vi "Main_DAQ.vi"() -> ()   [LabVIEW 2018]
uses:
  <vilib>/DAQmx/read.llb/DAQmx Read (Analog 2D DBL NChan NSamp).vi
  <vilib>/Analysis/baseanly.llb/Mean (DBL).vi
  <vilib>/DAQmx/create/channels.llb/DAQmx Create Channel (AI-Voltage-Basic).vi
  <vilib>/DAQmx/configure/timing.llb/DAQmx Timing (Sample Clock).vi
  <vilib>/DAQmx/configure/trigger.llb/DAQmx Start Trigger (Digital Edge).vi
  <vilib>/DAQmx/configure/trigger.llb/DAQmx Start Trigger (Time).vi
  <vilib>/DAQmx/configure/trigger.llb/DAQmx Start Trigger (Analog Edge).vi
  <vilib>/DAQmx/miscellaneous.llb/DAQmx Fill In Error Info.vi
  <resource>/objmgr/daqmx.rc
  <vilib>/Analysis/NI_AALBase.lvlib
panel:
  out "Waveform Graph 2":dbl[][](graph)
  out "Waveform Chart":dbl[](graph)
  in  "length":i32
  in  "Start index":i32
  in  "Path":path
  in  "Name File":string
  in  "SAVE ?":bool
  in  "SENSOR":bool
  in  "Trigger Type":T1(tab)=enum."Digital Start"
  in  "Digital Start Trigger Edge":i32(ring)=10280 caption="Edge" items=["Rising"=10280, "Falling"=10171]
  in  "Digital Start Trigger Source":tag="/Dev2/PFI0" caption="Source"
  in  "Digital Pause Trigger Pause When":i32(ring)=10192 caption="Pause When" items=["High"=10192, "Low"=10214]
  in  "Digital Pause Trigger Source":tag="/Dev1/PFI0" caption="Source"
  in  "Analog Start Trigger Level":dbl caption="Level" format="%0.2f"
  in  "Analog Start Trigger Hysteresis":dbl caption="Hysteresis" format="%.2f"
  in  "Analog Start Trigger Slope":i32(ring)=10280 caption="Slope" items=["Rising"=10280, "Falling"=10171]
  in  "Analog Start Trigger Source":string="APFI0" caption="Source"
  in  "Analog Pause Trigger Source":string="APFI0" caption="Source"
  in  "Analog Pause Trigger Pause When":i32(ring)=10093 caption="Pause When" items=["Above Level"=10093, "Below Level"=10107]
  in  "Analog Pause Trigger Level":dbl caption="Level" format="%.2f"
  in  "When":timestamp
  in  "Select Time\nManually":bool
  in  "Number of Samples":i32=100
  in  "Sample Rate":dbl=10000.0
  in  "Sample Clock Source":tag="OnboardClock"
  in  "Terminal Configuration":i32(ring)=10083 items=["default"=-1, "RSE"=10083, "NRSE"=10078, "Differential"=10106, "Pseudodifferential"=12529]
  in  "Max Voltage":dbl=10.0
  in  "Min Voltage":dbl=-10.0
  in  "Physical Channel":tag="Dev2/ai3:4"
  out "Actual Sample Rate":dbl=1000.0 format="%0.2f"
  # "Graph"
  # "Channel Settings"
  # "Control Program"
  # "Timing Settings"
  # "Saving Data Settings"
  # "Trigger Settings"
  # "To enable triggers, select a tab above, and configure the settings.\n\nNot all hardware supports all trigger types. Refer to your device documentation for more information."
  # "This trigger type is not supported in continuous sample timing. \n\nRefer to your device documentation for more information on which triggers are supported."
  # "This trigger type is not supported in continuous sample timing. \n\nRefer to your device documentation for more information on which triggers are supported."
  # "If time is not manually set, task will begin after 10 seconds"
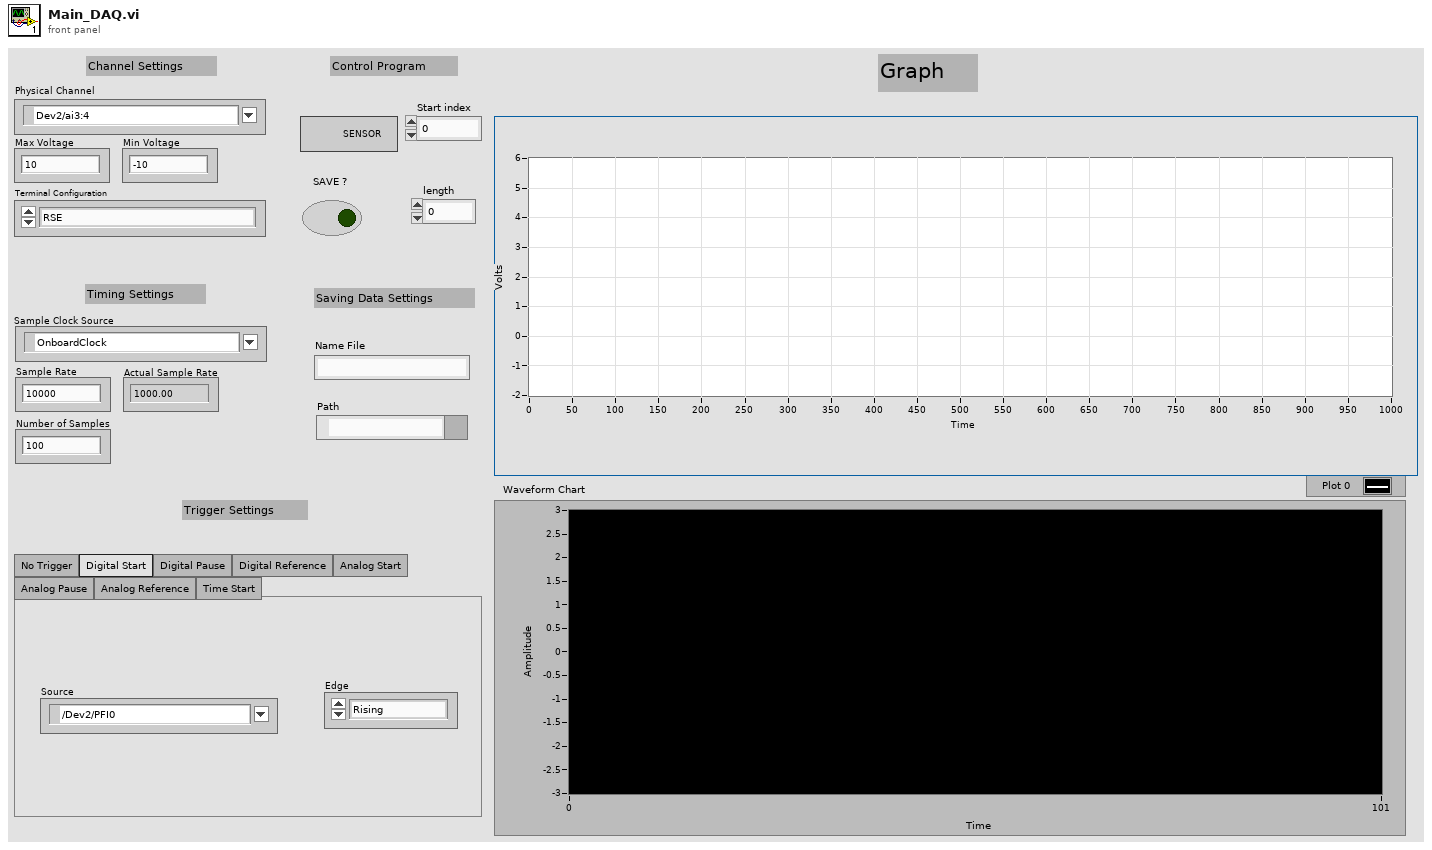
[diagram p1: front panel]
types:
  T1 = enum32{"No Trigger", "Digital Start", "Digital Pause", "Digital Reference", "Analog Start", "Analog Pause", "Analog Reference", "Time Start"}
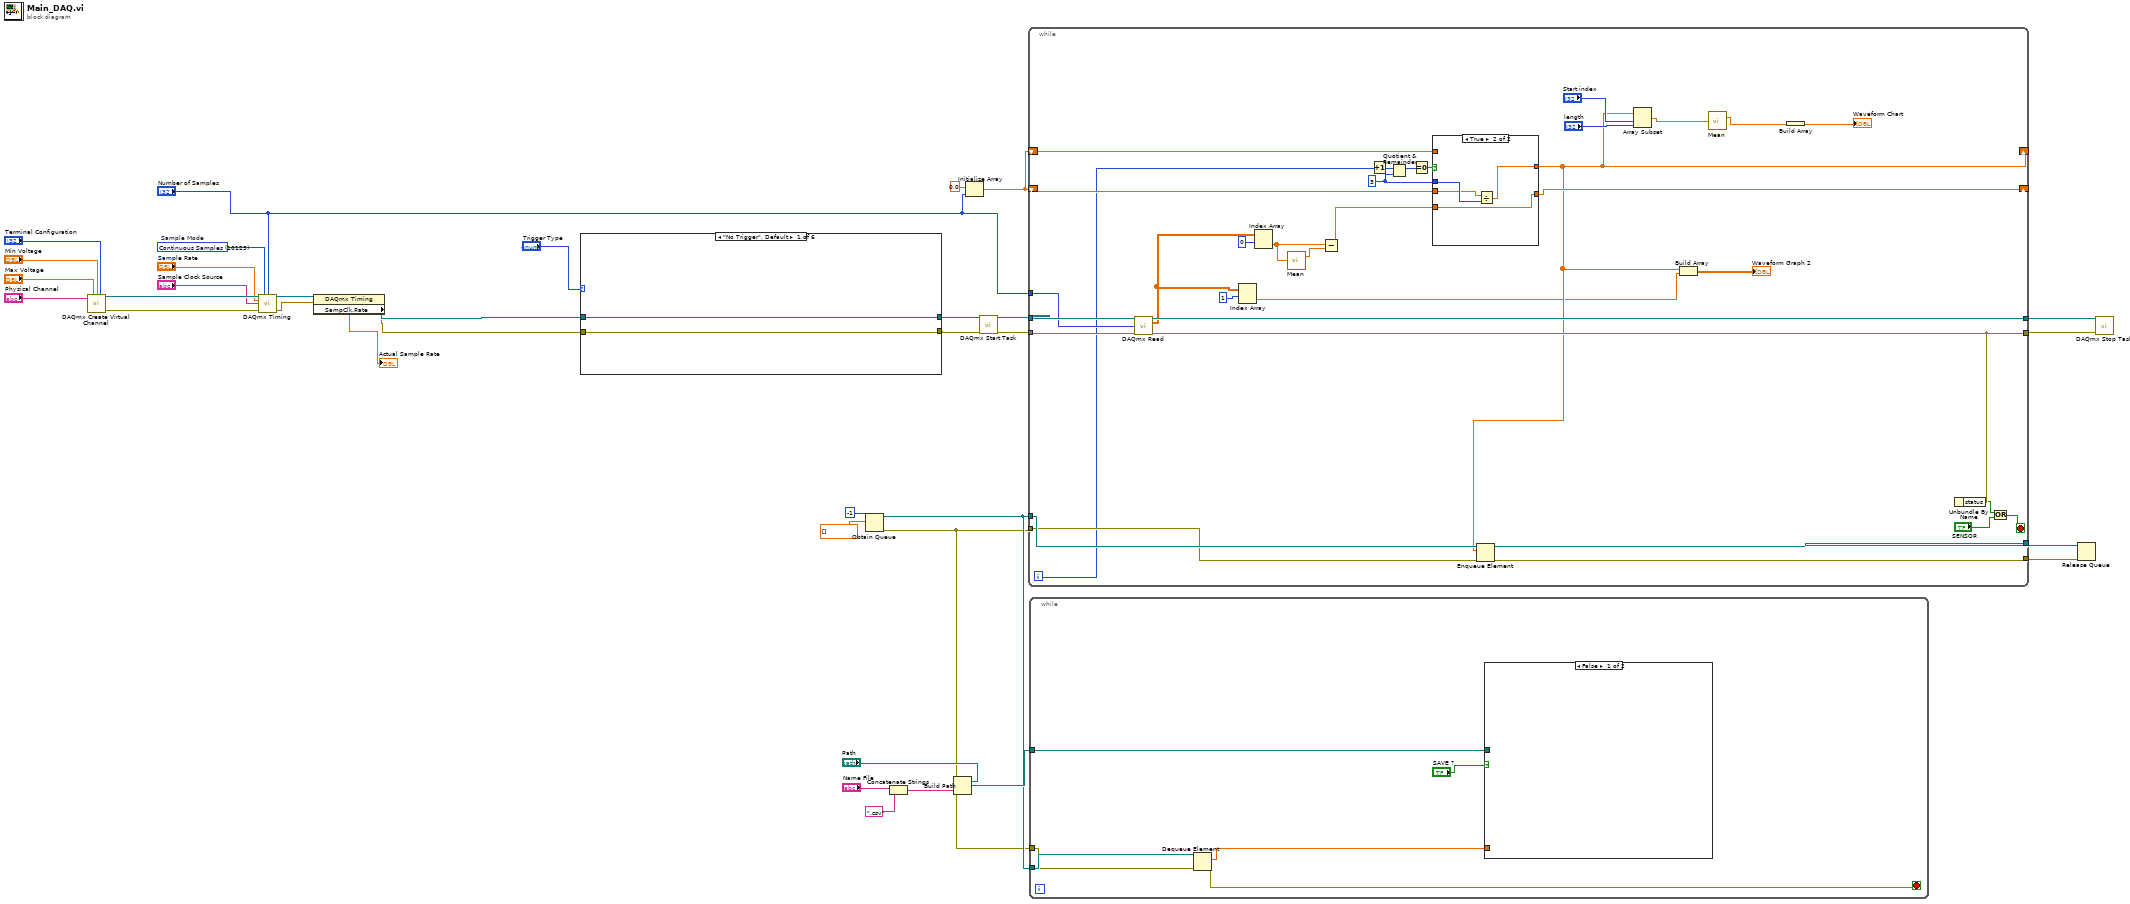
[diagram p0: block diagram]
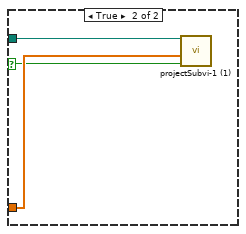
[diagram p2: hidden frame]
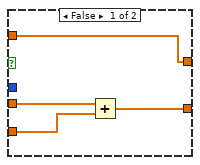
[diagram p3: hidden frame]
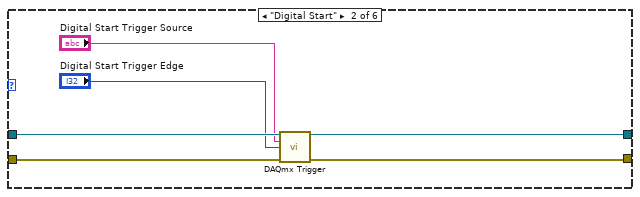
[diagram p4: hidden frame]
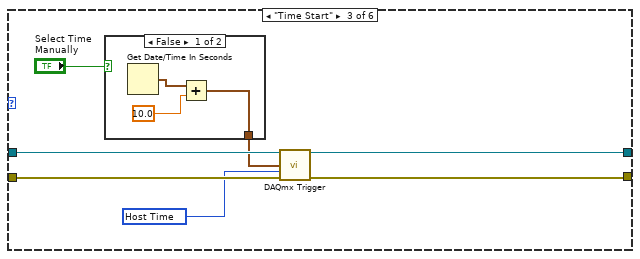
[diagram p5: hidden frame]
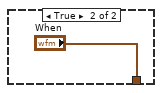
[diagram p6: hidden frame]
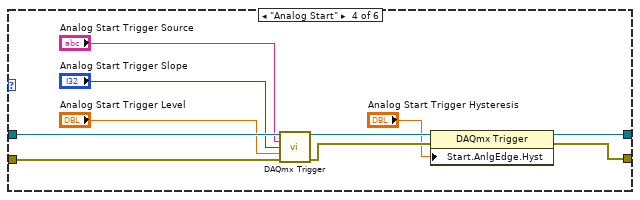
[diagram p7: hidden frame]
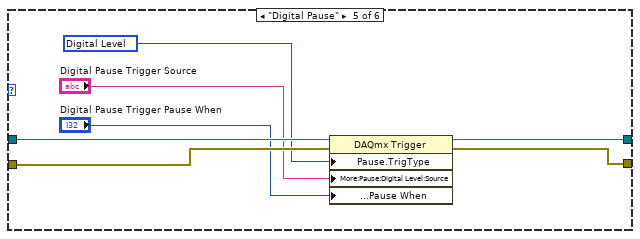
[diagram p8: hidden frame]
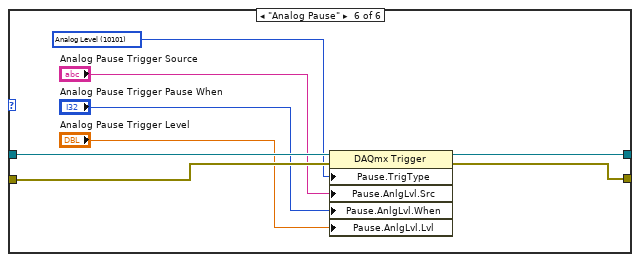
[diagram p9: hidden frame]
diagram:
  w33 = 10123 items=["Finite Samples"=10178, "Continuous Samples"=10123, "Hardware Timed Single Point"=12522]  # Sample Mode
  n1 = call-poly <vilib>:"DAQmx Create Virtual Channel.vi"("maximum value"="Max Voltage", "minimum value"="Min Voltage", "input terminal configuration"="Terminal Configuration", "physical channels"="Physical Channel") -> ("task out"=w31:refnum<k21>, "error out"=w32:errorcluster)  [unwired: 10 in]
  n2 = call-poly <vilib>:"DAQmx Timing.vi"("task/channels in"=w31, "sample mode"=w33, "samples per channel"="Number of Samples", "rate"="Sample Rate", "source"="Sample Clock Source", "error in"=w32) -> ("task out"=w35:refnum<k21>, "error out"=w34:errorcluster)  [unwired: 8 in]
  n3 = property class="DAQmx Timing"(reference=w35, error in=w34) -> (reference out=w20:refnum<k21>, error out=w19:errorcluster, "SampClk.Rate"=→"Actual Sample Rate":dbl)
  n4 = case shown="\"No Trigger\", Default" "Trigger Type" {
    tunnel: w20 -> [w37 w43 w50 w64 w71 w79]
    tunnel: w19 -> [w36 w42 w49 w63 w68 w76]
    tunnel: [w37 w41 w48 w61 w70 w78] -> w21
    tunnel: [w36 w40 w47 w60 w69 w77] -> w22
    frame "No Trigger", Default {
    }
    frame "Digital Start" {
      n5 = call-poly <vilib>:"DAQmx Trigger.vi"("task/channels in"=w43, "source"="Digital Start Trigger Source", "edge"="Digital Start Trigger Edge", "error in"=w42) -> ("task out"=w41:refnum<k21>, "error out"=w40:errorcluster)  [unwired: 10 in]
    }
    frame "Time Start" {
      w46 = 16126 items=["Host Time"=16126, "I/O Device Time"=16127] ("timescale")
      n6 = case shown="False" "Select Time\nManually" {
        tunnel: [w51 "When"] -> w44
        frame False {
          n7 = Get Date/Time In Seconds() -> (seconds since 1Jan1904=w53:timestamp)
          n8 = Add(x=w53, y=10.0) -> (x+y=w51:timestamp)
        }
        frame True {
        }
      }
      n9 = call-poly <vilib>:"DAQmx Trigger.vi"("task/channels in"=w50, "when"=w44, "timescale"=w46, "error in"=w49) -> ("task out"=w48:refnum<k21>, "error out"=w47:errorcluster)  [unwired: 10 in]
    }
    frame "Analog Start" {
      n10 = call-poly <vilib>:"DAQmx Trigger.vi"("task/channels in"=w64, "source"="Analog Start Trigger Source", "slope"="Analog Start Trigger Slope", "level"="Analog Start Trigger Level", "error in"=w63) -> ("task out"=w59:refnum<k21>, "error out"=w58:errorcluster)  [unwired: 9 in]
      n11 = property class="DAQmx Trigger"(reference=w59, error in=w58, "Start.AnlgEdge.Hyst"="Analog Start Trigger Hysteresis") -> (reference out=w61:refnum<k21>, error out=w60:errorcluster)
    }
    frame "Digital Pause" {
      w67 = 10152 items=["Analog Level"=10101, "Analog Window"=10103, "Digital Level"=10152, "Digital Pattern"=10398, "None"=10230] ("Pause.TrigType")
      n12 = property class="DAQmx Trigger"(reference=w71, error in=w68, "Pause.TrigType"=w67, "More:Pause:Digital Level:Source"="Digital Pause Trigger Source", "More:Pause:Digital Level:Pause When"="Digital Pause Trigger Pause When") -> (reference out=w70:refnum<k21>, error out=w69:errorcluster)
    }
    frame "Analog Pause" {
      w75 = 10101 items=["Analog Level"=10101, "Analog Window"=10103, "Digital Level"=10152, "Digital Pattern"=10398, "None"=10230] ("Pause.TrigType")
      n13 = property class="DAQmx Trigger"(reference=w79, error in=w76, "Pause.TrigType"=w75, "Pause.AnlgLvl.Src"="Analog Pause Trigger Source", "Pause.AnlgLvl.When"="Analog Pause Trigger Pause When", "Pause.AnlgLvl.Lvl"="Analog Pause Trigger Level") -> (reference out=w78:refnum<k21>, error out=w77:errorcluster)
    }
  }
  n14 = Obtain Queue(max queue size (-1, unlimited)=-1, element data type=dbl[] [] ("Radar output")) -> (queue out=w7:refnum<queue>, error out=w4:errorcluster)  [unwired: 3 in, 1 out]
  n15 = Concatenate Strings("Name File", ".csv" ("string")) -> (w12:string)
  n16 = Build Path(base path="Path", name or relative path=w12) -> (appended path=w10:path)
  n17 = Initialize Array(0.0 ("element"), "Number of Samples") -> (w1:dbl[])
  n18 = call <vilib>:"DAQmx Start Task.vi"("task/channels in"=w21, "error in"=w22) -> ("task out"=w16:refnum<k21>, "error out"=w15:errorcluster)  [unwired: 12 in]
  n19 = while {
    tunnel: w16 -> [w113]
    tunnel: w15 -> [w112]
    tunnel: [w111] -> w18
    tunnel: [w109] -> w17
    tunnel: "Number of Samples" -> [w107]
    tunnel: w7 -> [w104]
    tunnel: w4 -> [w103]
    tunnel: [w102] -> w6
    tunnel: [w101] -> w5
    shift-right: [w97] -> _
    shift-left: w1 -> [w99]
    shift-right: [w81] -> _
    shift-left: w1 -> [w91]
    i -> [w96]
    stop <- w105 stop-if-true
    w92 = 3 ("y")
    n20 = call-poly <vilib>:"DAQmx Read.vi"("task/channels in"=w113, "number of samples per channel"=w107, "error in"=w112) -> ("task out"=w111:refnum<k21>, "data"=w83:dbl[][], "error out"=w109:errorcluster)  [unwired: 10 in]
    n21 = Index Array(array=w83, index (row)=1) -> (element=w80:dbl[])  [unwired: 1 in]
    n22 = Index Array(array=w83, index (row)=0) -> (element=w90:dbl[])  [unwired: 1 in]
    n23 = call-poly <vilib>:"Mean.vi"("X"=w90) -> ("mean"=w100:dbl)  [unwired: 1 out]
    n24 = Subtract(x=w90, y=w100) -> (x-y=w98:dbl[])
    n25 = Increment(x=w96) -> (x+1=w95:i32)
    n26 = Quotient & Remainder(x=w95, y=w92) -> (x-y*floor(x/y)=w94:i32)  [unwired: 1 out]
    n27 = Equal To 0?(x=w94) -> (x = 0?=w93:bool)
    n28 = case shown="True" w93 {
      tunnel: w99 -> [w117 w120]
      tunnel: w98 -> [w116 w118]
      tunnel: [w115 w118] -> w97
      tunnel: w92 -> [_ w121]
      tunnel: [w114 w119] -> w81
      tunnel: w91 -> [w114 _]
      frame False {
        n29 = Add(x=w117, y=w116) -> (x+y=w115:dbl[])
      }
      frame True {
        n30 = Divide(x=w120, y=w121) -> (x/y=w119:dbl[])
      }
    }
    n31 = Enqueue Element(queue=w104, element=w81, error in (no error)=w103) -> (queue out=w102:refnum<queue>, error out=w101:errorcluster)  [unwired: 1 in, 1 out]
    n32 = Array Subset(array=w81, index="Start index", length="length") -> (w87:dbl[])
    n33 = Build Array(w81, w80) -> (→"Waveform Graph 2":dbl[][])
    n34 = call-poly <vilib>:"Mean.vi"("X"=w87) -> ("mean"=w86:dbl)  [unwired: 1 out]
    n35 = Build Array(w86) -> (→"Waveform Chart":dbl[])
    n36 = Unbundle By Name(w109) -> ("status"=w108:bool)
    n37 = Or(x=w108, y="SENSOR") -> (x .or. y?=w105:bool)
  }
  n38 = while {
    tunnel: w4 -> [w123]
    tunnel: w7 -> [w124]
    tunnel: w10 -> [w125]
    stop <- w127 stop-if-true
    n39 = Dequeue Element(queue=w124, error in (no error)=w123) -> (element=w122:dbl[], error out=w127:errorcluster)  [unwired: 1 in, 2 out]
    n40 = case shown="False" "SAVE ?" {
      selector: "SAVE ?" -> [_ w128]
      tunnel: w122 -> [_ w129]
      tunnel: w125 -> [_ w130]
      frame False {
      }
      frame True {
        n41 = call "projectSubvi-1 (1).vi"("append to file? (new file:F)"=w128, "1D data"=w129, "file path (dialog if empty)"=w130) -> ()  [unwired: 9 in]
      }
    }
  }
  n42 = Release Queue(queue=w6, error in (no error)=w5) -> ()  [unwired: 1 in, 3 out]
  n43 = call <vilib>:"DAQmx Stop Task.vi"("task/channels in"=w18, "error in"=w17) -> ()  [unwired: 12 in, 2 out]
